vi "Actor-Caller Proxy.vi"(5 "Initialize-Error Passback":refnum<notifier>, 7 "Enqueuers Passback":refnum<notifier>, 8 "Owner":refnum<vi>, 9 "Stopped Enqueuer":refnum<user-event>, 10 "Launch":refnum<notifier>, 11 "Actor in":refnum<class "Actor.lvclass">) -> ()   [LabVIEW 2018]
uses:
  Interface.lvclass
  Actor.lvclass
  State.ctl
  Get State.ctl
  Stop.ctl
  Request-Enqueuers.ctl
  Stopped.ctl
  Front-Panel State.ctl
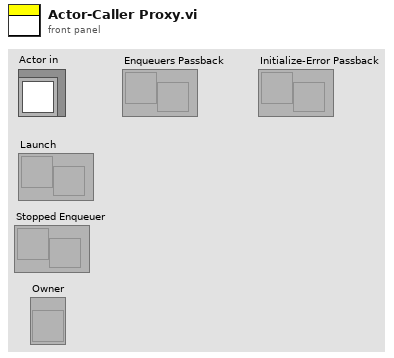
[diagram p1: front panel]
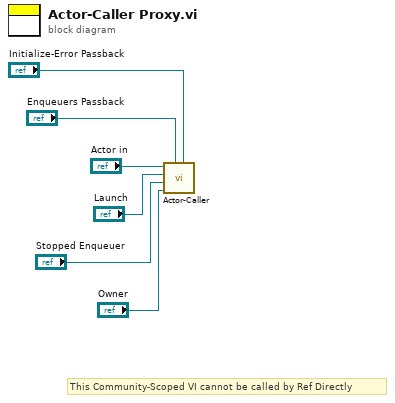
[diagram p0: block diagram]
diagram:
  # "This Community-Scoped VI cannot be called by Ref Directly"
  n1 = call "Actor-Caller.vi"("Initialize-Error Passback"="Initialize-Error Passback", "Enqueuers Passback"="Enqueuers Passback", "Owner"="Owner", "Stopped Enqueuer"="Stopped Enqueuer", "Launch"="Launch", "Actor in"="Actor in") -> ()  [unwired: 6 in]
